vi "ABR-Restore Defaults.vi"() -> (4 "Params":T5={"CAP or ABR"=enum."ABR", "Stimulus"={"Ear"=enum."Left", "Start (dB)"=0, "Waveform"=enum."TONE PIP", "Stop (dB)"=30, "Frequency (kHz)"=16.0, "Step (dB)"=5, "Rep rate (/sec)"=30.0, "Alternate Polarity"=FALSE}, "Response"={"Gain"=10000, "Averages"=512, "Window (ms)"=8.5, "Thr Fast Steps"=8.5}, "Hidden"={"AI Samp Rate Hz"=25000.0, "AO Samp Rate Hz"=100000.0, "Duration (ms)"=5.0, "Ramp (ms)"=0.5, "Click width (us)"=100.0, "ITI"=enum."Rate", "Save raw"=FALSE}, "Version"=0} {"Response"."Thr Fast Steps" format="%.2f"; "Response"."Window (ms)" format="%.2f"; "Stimulus"."Frequency (kHz)" format="%.2f"; "Stimulus"."Start (dB)" step=5}, 8 "Threshold Estimation":T1={"Tmin (ms)"=0.0, "Tmax (ms)"=8.5, "CC criterion"=0.35, "adjR2 criterion"=0.7}, 15 "error out":errorcluster)   [LabVIEW 2020]
uses:
  TypeDefs/ABR-Parameters.ctl
  TypeDefs/ABR-Stimulus.ctl
  TypeDefs/ABR-Response.ctl
  TypeDefs/ABR-Hidden Params.ctl
  Threshold Estimation VIs/ABR3-Threshold Estimation Parameters.ctl
panel:
  in  "Hidden":T2={"AI Samp Rate Hz"=25000.0, "AO Samp Rate Hz"=100000.0, "Duration (ms)"=5.0, "Ramp (ms)"=0.5, "AO Npts"=0, "AI Npts"=0, "AI Offset"=0, "Click width (us)"=0.0}
  in  "Response":T3={"Gain"=10000, "Averages"=512, "Window (ms)"=8.5, "Thr Fast Steps"=8.5} {"Thr Fast Steps" format="%.2f"; "Window (ms)" format="%.2f"}
  in  "CAP or ABR":enum16{"CAP", "ABR"}(ring)=enum."ABR" caption="Measure what"
  in  "Stimulus":T4={"Ear"=enum."Left", "Start (dB)"=20, "Waveform"=enum."TONE PIP", "Stop (dB)"=80, "Frequency (kHz)"=16.0, "Step (dB)"=5, "Rep rate (/sec)"=30.0, "Alternate Polarity"=FALSE} {"Frequency (kHz)" format="%.2f"; "Start (dB)" step=5}
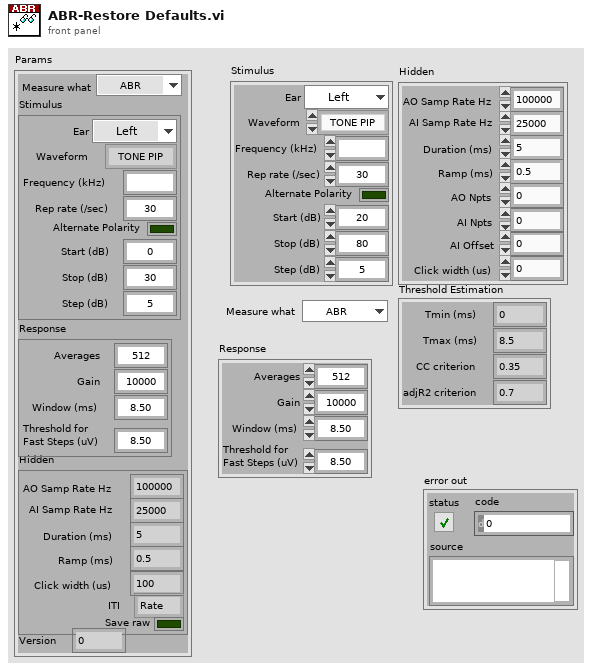
[diagram p1: front panel]
types:
  T1 = typedef "ABR3-Threshold Estimation Parameters.ctl" = cluster{"Tmin (ms)":dbl, "Tmax (ms)":dbl, "CC criterion":dbl, "adjR2 criterion":dbl}
  T2 = cluster{"AI Samp Rate Hz":dbl, "AO Samp Rate Hz":dbl, "Duration (ms)":dbl, "Ramp (ms)":dbl, "AO Npts":i32, "AI Npts":i32, "AI Offset":i32, "Click width (us)":dbl}
  T3 = typedef "ABR-Response.ctl" = cluster{"Gain":i32, "Averages":i32, "Window (ms)":sgl, "Thr Fast Steps":sgl}
  T4 = typedef "ABR-Stimulus.ctl" = cluster{"Ear":enum16{"Right", "Left", "Bone"}, "Start (dB)":i32, "Waveform":enum16{"TONE PIP", "CLICK"}, "Stop (dB)":i32, "Frequency (kHz)":ext, "Step (dB)":i32, "Rep rate (/sec)":dbl, "Alternate Polarity":bool}
  T5 = typedef "ABR-Parameters.ctl" = cluster{"CAP or ABR":enum16{"CAP", "ABR"}, "Stimulus":T4, "Response":T3, "Hidden":T6, "Version":i32}
  T6 = typedef "ABR-Hidden Params.ctl" = cluster{"AI Samp Rate Hz":dbl, "AO Samp Rate Hz":dbl, "Duration (ms)":dbl, "Ramp (ms)":dbl, "Click width (us)":dbl, "ITI":enum16{"Rate", "Interval"}, "Save raw":bool}
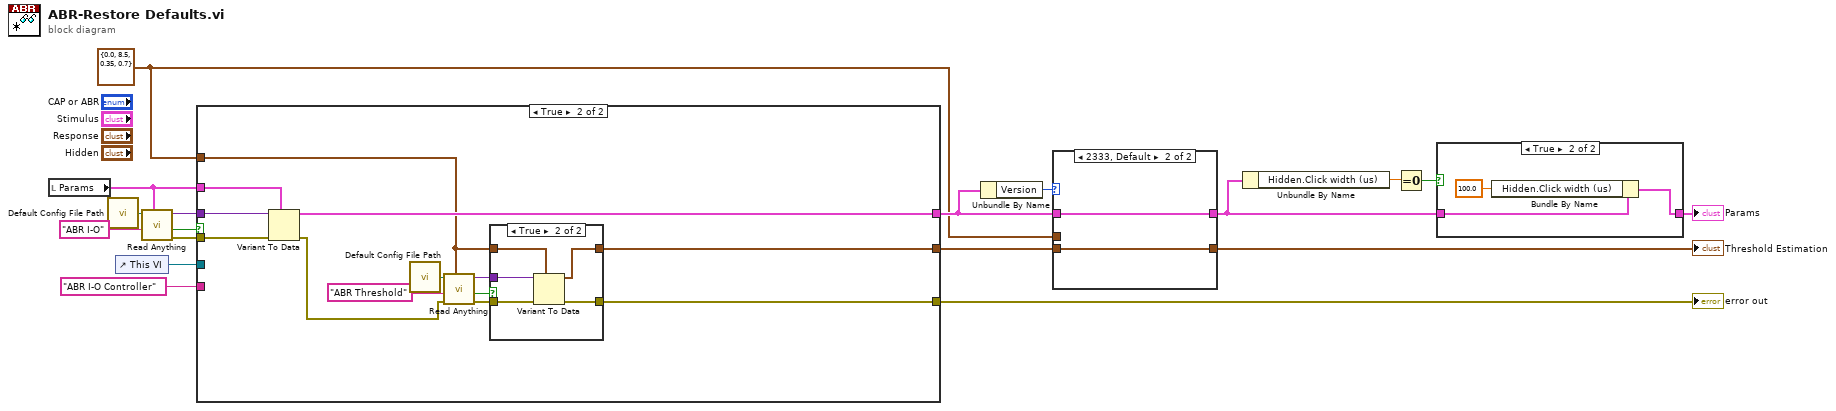
[diagram p0: block diagram]
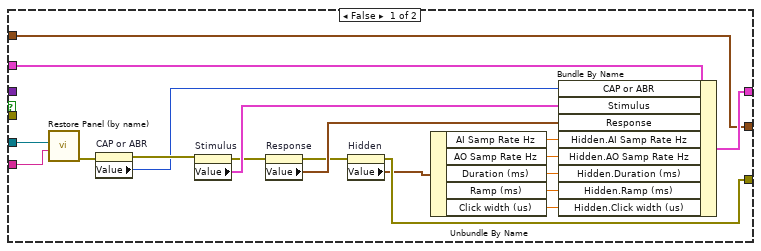
[diagram p4: hidden frame]
diagram:
  w5 = T1 {"Tmin (ms)"=0.0, "Tmax (ms)"=8.5, "CC criterion"=0.35, "adjR2 criterion"=0.7} ("Threshold Estimation")
  n1 = local read "Params"() -> (w16:T5)
  n2 = call "Default Config File Path.vi"() -> ("Default config file name"=w17:path)
  n3 = control-ref of="This VI"() -> (w12:refnum<vi>)
  n4 = call "Read Anything.vi"("Type of Anything"=w16, "Section Name (Name of \"Type of Anything\")"="ABR I-O" ("Section Name (Name of \"Type of Anything\")"), "Path (dialog)"=w17) -> ("Error Out"=w14:errorcluster, "Found?"=w13:bool, "Anything"=w18:variant)  [unwired: 6 in]
  n5 = case shown="True" w13 {
    tunnel: w18 -> [_ w50]
    tunnel: w16 -> [w37 w49]
    tunnel: w14 -> [_ w48]
    tunnel: w12 -> [w34 _]
    tunnel: [w36 w47] -> w8
    tunnel: "ABR I-O Controller" ("Section Name (Name of \"Type of Anything\")") -> [w33 _]
    tunnel: [w26 w39] -> w10
    tunnel: [w19 w40] -> w6
    tunnel: w5 -> [w19 w38]
    frame False {
      n6 = call "Restore Panel (by name).vi"("Name"=w33, "VI reference"=w34) -> ("error out"=w32:errorcluster)  [unwired: 9 in]
      n7 = property on="CAP or ABR" class="Enum (strict)"(error in=w32) -> (error out=w31:errorcluster, "Value"=w30:enum16{"CAP", "ABR"})  [unwired: 1 in, 1 out]
      n8 = property on="Stimulus" class="Clust (strict)"(error in=w31) -> (error out=w29:errorcluster, "Value"=w35:T4)  [unwired: 1 in, 1 out]
      n9 = property on="Response" class="Clust (strict)"(error in=w29) -> (error out=w27:errorcluster, "Value"=w28:T3)  [unwired: 1 in, 1 out]
      n10 = property on="Hidden" class="Clust (strict)"(error in=w27) -> (error out=w26:errorcluster, "Value"=w25:T2)  [unwired: 1 in, 1 out]
      n11 = Unbundle By Name(w25) -> ("AI Samp Rate Hz"=w24:dbl, "AO Samp Rate Hz"=w23:dbl, "Duration (ms)"=w22:dbl, "Ramp (ms)"=w21:dbl, "Click width (us)"=w20:dbl)
      n12 = Bundle By Name(cluster=w37, "CAP or ABR"=w30, "Stimulus"=w35, "Response"=w28, "Hidden.AI Samp Rate Hz"=w24, "Hidden.AO Samp Rate Hz"=w23, "Hidden.Duration (ms)"=w22, "Hidden.Ramp (ms)"=w21, "Hidden.Click width (us)"=w20) -> (w36:T5)
    }
    frame True {
      n13 = Variant To Data(error in=w48, type=w49, Variant=w50) -> (data=w47:T5, error out=w44:errorcluster)
      n14 = call "Default Config File Path.vi"() -> ("Default config file name"=w46:path)
      n15 = call "Read Anything.vi"("Type of Anything"=w38, "Error In"=w44, "Section Name (Name of \"Type of Anything\")"="ABR Threshold" ("Section Name (Name of \"Type of Anything\")"), "Path (dialog)"=w46) -> ("Error Out"=w41:errorcluster, "Found?"=w43:bool, "Anything"=w42:variant)  [unwired: 5 in]
      n16 = case shown="True" w43 {
        tunnel: w42 -> [_ w56]
        tunnel: w38 -> [w52 w55]
        tunnel: w41 -> [w51 w57]
        tunnel: [w52 w54] -> w40
        tunnel: [w51 w53] -> w39
        frame False {
        }
        frame True {
          n17 = Variant To Data(error in=w57, type=w55, Variant=w56) -> (data=w54:T1, error out=w53:errorcluster)
        }
      }
    }
  }
  "error out" <- w10
  n18 = Unbundle By Name(w8) -> ("Version"=w9:i32)
  n19 = case shown="2333, Default" w9 {
    tunnel: [w58 w61] -> w2
    tunnel: w8 -> [w58 w61]
    tunnel: [w59 w60] -> w7
    tunnel: w6 -> [_ w60]
    tunnel: w5 -> [w59 _]
    frame 0..2332 {
    }
    frame 2333, Default {
    }
  }
  "Threshold Estimation" <- w7
  n20 = Unbundle By Name(w2) -> ("Hidden.Click width (us)"=w4:dbl)
  n21 = Equal To 0?(x=w4) -> (x = 0?=w3:bool)
  n22 = case shown="True" w3 {
    tunnel: w2 -> [w62 w65]
    tunnel: [w62 w63] -> w1
    frame False {
    }
    frame True {
      n23 = Bundle By Name(cluster=w65, "Hidden.Click width (us)"=100.0) -> (w63:T5)
    }
  }
  "Params" <- w1
